vi "Delacor_lib_QMH_Flush Messages.vi"(8 "error in":errorcluster, 11 "Message Queue in":refnum<class "ModuleQueue.lvclass">) -> (0 "error out":errorcluster, 1 "Remaining Message Data":variant[](array[variant]), 2 "Remaining Messages":string[](array[string]), 3 "Message Queue out":refnum<class "ModuleQueue.lvclass">)   [LabVIEW 2024, in "ModuleQueue.lvclass"]
doc: "Flush the message queue.\n____\nDQMH Framework: Palette 7.1.0.1503\nCopyright (c) 2025, DQMH Consortium"
uses:
  ModuleQueue.lvclass
  ModuleQueue.lvclass/ModuleQueue.ctl
  Delacor_lib_QMH_Get Message Queue.vi
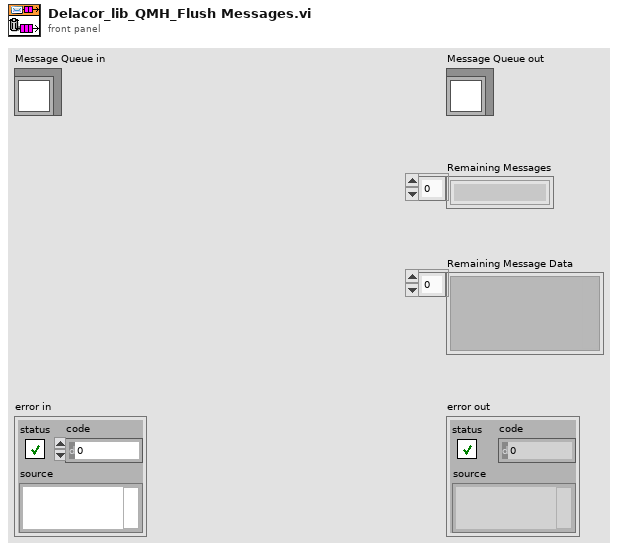
[diagram p1: front panel]
types:
  T1 = typedef "ModuleQueue.lvclass/Delacor_lib_QMH_Message--cluster.ctl" = cluster{"Message":string, "Message Data":variant}
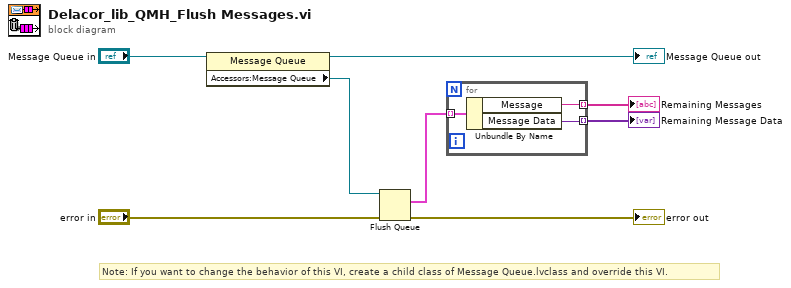
[diagram p0: block diagram]
diagram:
  # "Note: If you want to change the behavior of this VI, create a child class of Message Queue.lvclass and override this VI."
  n1 = property class="Message Queue"(reference="Message Queue in") -> (reference out=→"Message Queue out":refnum<class "ModuleQueue.lvclass">, "Accessors:Message Queue"=w5:refnum<queue>)  [unwired: 1 in, 1 out]
  n2 = Flush Queue(queue=w5, error in (no error)="error in") -> (remaining elements=w3:T1[], error out=→"error out":errorcluster)  [unwired: 1 out]
  n3 = for {
    tunnel: w3 -> [w11] mode=indexing
    tunnel: [w10] -> w2 mode=indexing
    tunnel: [w9] -> w1 mode=indexing
    n4 = Unbundle By Name(w11) -> ("Message"=w10:string, "Message Data"=w9:variant)
  }
  "Remaining Messages" <- w2
  "Remaining Message Data" <- w1
